vi "时间重合区间.vi"(11 "曲线":cluster{"时间":dbl[], "力":dbl[]}[](array[cluster])) -> (2 "最小值":dbl, 3 "最大值":dbl)   [LabVIEW 2015]
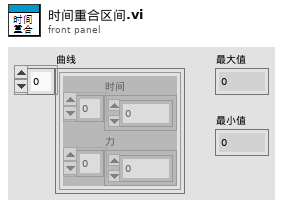
[diagram p1: front panel]
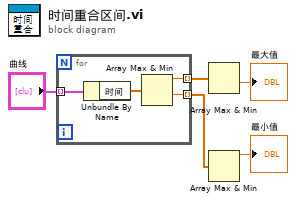
[diagram p0: block diagram]
diagram:
  n1 = for {
    tunnel: "曲线" -> [w9] mode=indexing
    tunnel: [w7] -> w2 mode=indexing
    tunnel: [w6] -> w3 mode=indexing
    n2 = Unbundle By Name(w9) -> ("时间"=w8:dbl[])
    n3 = Array Max & Min(array=w8) -> (max value=w7:dbl, min value=w6:dbl)  [unwired: 2 out]
  }
  n4 = Array Max & Min(array=w2) -> (min value=→"最大值":dbl)  [unwired: 3 out]
  n5 = Array Max & Min(array=w3) -> (max value=→"最小值":dbl)  [unwired: 3 out]
